vi "cw_2_2.vi"() -> ()   [LabVIEW 2022 SP3]
uses:
  <vilib>/numeric/Random Number (Range) I64.vi
  <vilib>/numeric/sub_Random U32.vi
panel:
  in  "y":bool
  out "discrimination level":bool
  in  "discrimination level":dbl=1.5 step=0.1
  in  "noise amplitude":dbl=0.5 step=0.1
  in  "frequency":dbl=2.0
  out "time":dbl
  out "Waveform Chart":cluster{dbl, "discrimination level":dbl}(graph)
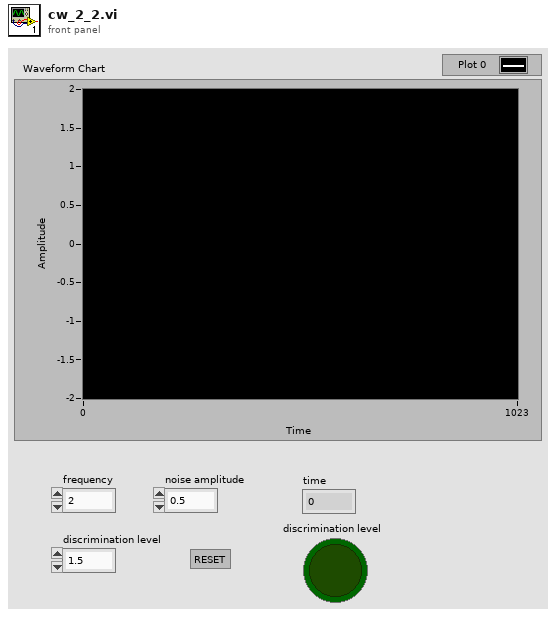
[diagram p1: front panel]
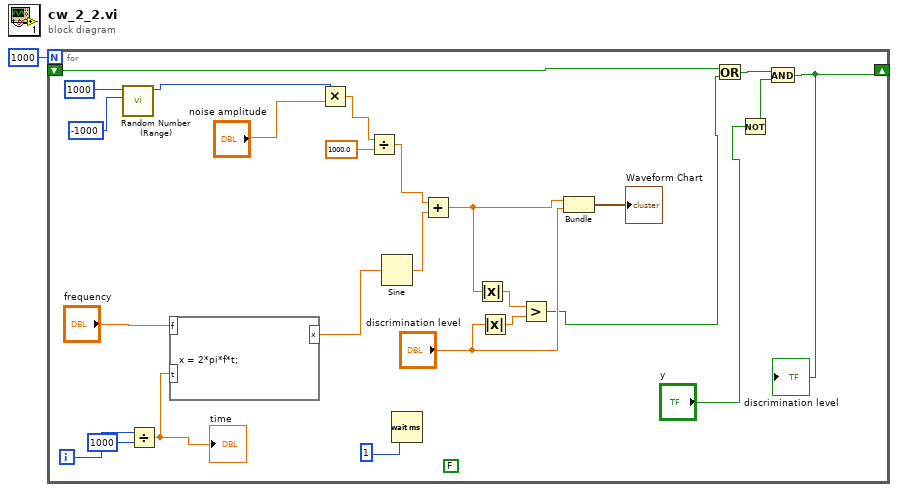
[diagram p0: block diagram]
diagram:
  n1 = for {
    N: 1000 -> [_]
    shift-right: [w4] -> _
    shift-left: _ -> [w6]
    i -> [w26]
    (unwired) FALSE
    n2 = call-poly <vilib>:"Random Number (Range).vi"("lower bound (-100)"=i64 -1000, "upper bound (100)"=i64 1000) -> ("number"=w16:i64)  [unwired: 9 in]
    n3 = Divide(x=w26, y=1000) -> (x/y=w23:dbl)
    "time" <- w23
    n4 = formula code="x = 2*pi*f*t;"("f"="frequency", "t"=w23) -> ("x"=w24:dbl)
    n5 = Multiply(x=w16, y="noise amplitude") -> (x*y=w15:dbl)
    n6 = Divide(x=w15, y=1000.0) -> (x/y=w14:dbl)
    n7 = Sine(x=w24) -> (sin(x)=w19:dbl)
    n8 = Wait (ms)(milliseconds to wait=u32 1) -> ()  [unwired: 1 out]
    n9 = Add(x=w14, y=w19) -> (x+y=w11:dbl)
    n10 = Absolute Value(x=w11) -> (abs(x)=w9:dbl)
    n11 = Absolute Value(x="discrimination level") -> (abs(x)=w8:dbl)
    n12 = Greater?(x=w9, y=w8) -> (0:w7:bool)
    n13 = Bundle(w11, "discrimination level"="discrimination level") -> (→"Waveform Chart":cluster{dbl, "discrimination level":dbl})  [unwired: 1 in]
    n14 = Or(x=w6, y=w7) -> (x .or. y?=w5:bool)
    n15 = Not(x="y") -> (.not. x?=w2:bool)
    n16 = And(x=w5, y=w2) -> (x .and. y?=w4:bool)
    "discrimination level" <- w4
  }
